vi "Scale Controls.vi"(7 "rules":string, 8 "error in (no error)":errorcluster, 9 "pane size":T3, 10 "Decorations on Pane":refnum<vi>[](array[refnum]), 11 "Controls on Pane":refnum<vi>[](array[refnum])) -> (0 "error out":errorcluster)   [LabVIEW 2020]
doc: "Simple and schmutzig VI that will scale controls and labeled decorations by delta change of pane size.\nUsage: put in multiline string with rules:\nmy control name a [edge:LRTB]\nmy control name b [edge:LRB]\n...\n\nwhere edge:LRTB defines edges to be sticked to pane. LR - scale horizontaly, R - no scale, move object only, TB - scale vertically, B - just stick object to bottom, no scaling...\nWhen using for decorations, name them first with script 'Set Decoration Label'!"
uses:
  <vilib>/Utility/miscctls.llb/LVRectTypeDef.ctl
  Scale Controls List.ctl
  Scale Controls Record.ctl
  <vilib>/regexp/Match Regular Expression.xnode
panel:
  in  "lists":T1[](array[typedef])
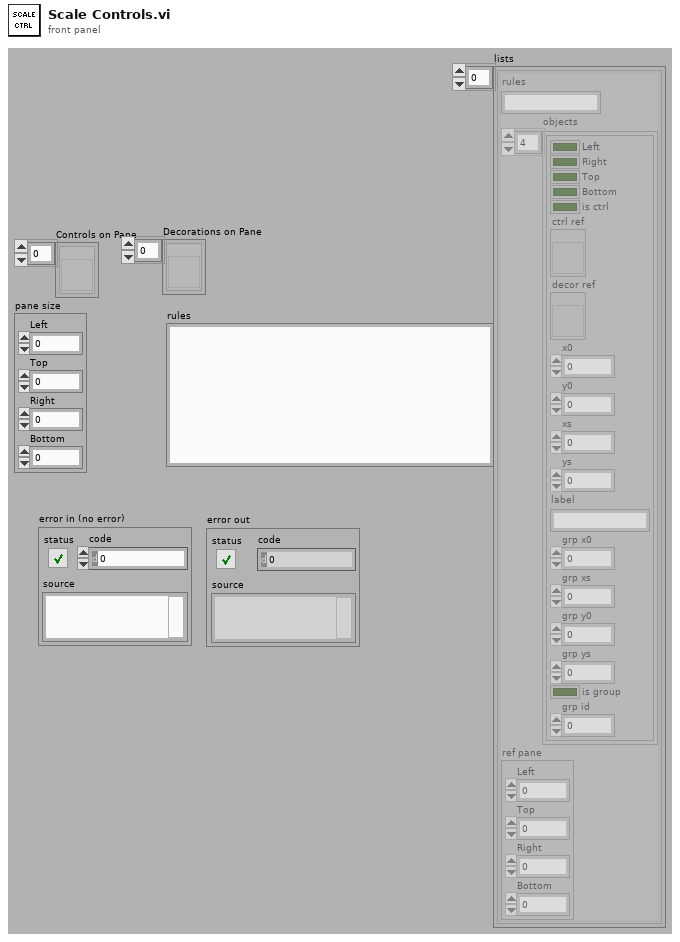
[diagram p1: front panel]
types:
  T1 = typedef "Scale Controls List.ctl" = cluster{"rules":string, "objects":T2[], "ref pane":T3}
  T2 = typedef "Scale Controls Record.ctl" = cluster{"Left":bool, "Right":bool, "Top":bool, "Bottom":bool, "is ctrl":bool, "ctrl ref":refnum<vi>, "decor ref":refnum<vi>, "x0":i32, "y0":i32, "xs":i32, "ys":i32, "label":string, "grp x0":i32, "grp xs":i32, "grp y0":i32, "grp ys":i32, "is group":bool, "grp id":i32}
  T3 = typedef "LVRectTypeDef.ctl" = cluster{"Left":i16, "Top":i16, "Right":i16, "Bottom":i16}
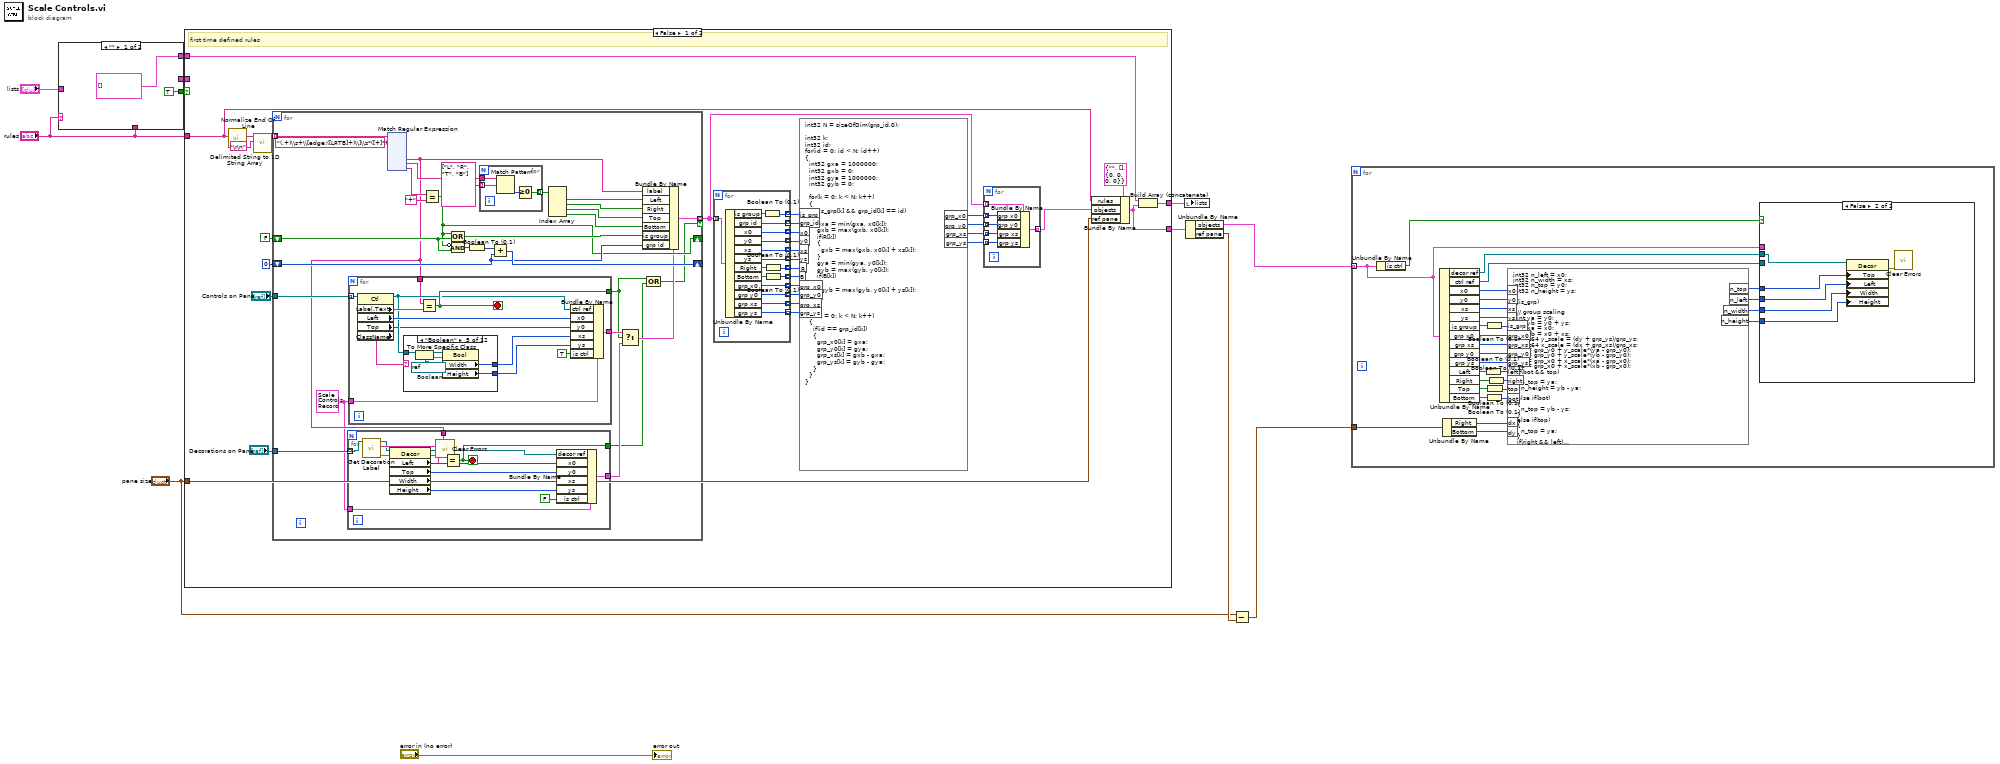
[diagram p0: block diagram]
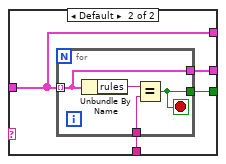
[diagram p2: hidden frame]
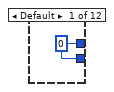
[diagram p3: hidden frame]
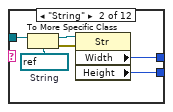
[diagram p4: hidden frame]
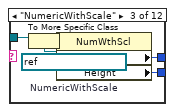
[diagram p5: hidden frame]
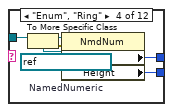
[diagram p6: hidden frame]
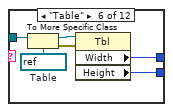
[diagram p7: hidden frame]
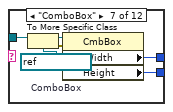
[diagram p8: hidden frame]
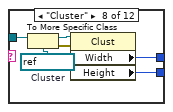
[diagram p9: hidden frame]
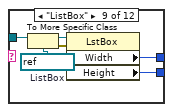
[diagram p10: hidden frame]
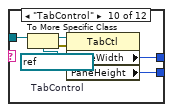
[diagram p11: hidden frame]
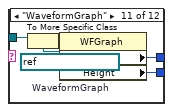
[diagram p12: hidden frame]
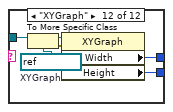
[diagram p13: hidden frame]
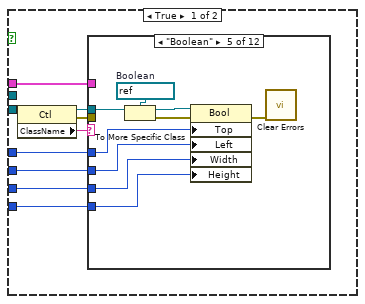
[diagram p15: hidden frame]
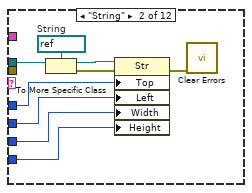
[diagram p17: hidden frame]
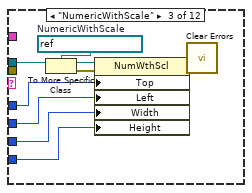
[diagram p18: hidden frame]
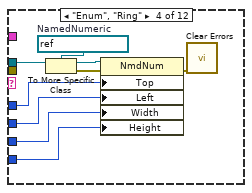
[diagram p19: hidden frame]
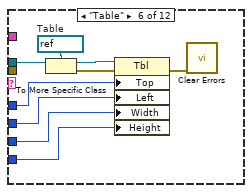
[diagram p20: hidden frame]
diagram:
  n1 = case shown="\"\"" "rules" {
    tunnel: [TRUE w18] -> w11
    tunnel: [_ w17] -> w9
    tunnel: "rules" -> [_ w16]
    tunnel: [T1[] [] ("lists") w15] -> w7
    tunnel: "lists" -> [_ w15]
    frame "" {
    }
    frame Default {
      n2 = for {
        tunnel: w15 -> [w19] mode=indexing
        tunnel: w16 -> [w21]
        tunnel: [w20] -> w18
        tunnel: [w19] -> w17
        stop <- w20 stop-if-true
        n3 = Unbundle By Name(w19) -> ("rules"=w22:string)
        n4 = Equal?(x=w22, y=w21) -> (x = y?=w20:bool)
      }
    }
  }
  n5 = case shown="False" w11 {
    tunnel: "rules" -> [w48 _]
    tunnel: w7 -> [w47 w322]
    tunnel: [w46 w322] -> w10
    tunnel: [w45 w323] -> w8
    tunnel: w9 -> [_ w323]
    tunnel: "pane size" -> [w44 _]
    frame False {
      # "first time defined rules"
      n6 = call <vilib>:"Normalize End Of Line.vi"("string in"=w48) -> ("string out"=w51:string)  [unwired: 7 in]
      n7 = call <vilib>:"Delimited String to 1D String Array.vi"("delimiter"="\r\n", "delimited string"=w51) -> ("string array"=w52:string[])  [unwired: 9 in]
      n8 = for {
        tunnel: w52 -> [w104] mode=indexing
        tunnel: [w94] -> w30 mode=indexing if=w76
        tunnel: "Controls on Pane" -> [w95]
        shift-right: [w85] -> _
        shift-left: FALSE -> [w91]
        shift-right: [w88] -> _
        shift-left: 0 -> [w87]
        tunnel: "Decorations on Pane" -> [w84]
        w82 = T2 {"Left"=FALSE, "Right"=FALSE, "Top"=FALSE, "Bottom"=FALSE, "is ctrl"=FALSE, "ctrl ref"=refnum, "decor ref"=refnum, "x0"=0, "y0"=0, "xs"=0, "ys"=0, "label"="", "grp x0"=0, "grp xs"=0, "grp y0"=0, "grp ys"=0, "is group"=FALSE, "grp id"=0} ("object")
        n9 = xnode "Match Regular Expression"("input string"=w104, "regular expression"="(.+)\\s+\\[edge:([LRTB]+)\\]\\s*([+]*)") -> ("submatch 1"=w83:string, "submatch 2"=w102:string, "submatch 3"=w93:string)  [unwired: 4 in, 5 out]
        n10 = for {
          tunnel: w84 -> [w108] mode=indexing
          tunnel: w83 -> [w115]
          tunnel: w82 -> [w114]
          tunnel: [w117] -> w80
          tunnel: [w116] -> w77
          stop <- w116 stop-if-true
          n11 = call "Get Decoration Label.vi"("Decor Refnum"=w108) -> ("error out"=w109:errorcluster, "Label"=w110:string, "dup Decor Refnum"=w107:refnum<vi>)  [unwired: 4 in]
          n12 = property class="Decor"(reference=w107, error in=w109) -> (reference out=w106:refnum<vi>, error out=w105:errorcluster, "Left"=w119:i32, "Top"=w113:i32, "Width"=w112:u32, "Height"=w111:u32)
          n13 = call <vilib>:"Clear Errors.vi"("error in (no error)"=w105) -> ()  [unwired: 5 in, 2 out]
          n14 = Equal?(x=w115, y=w110) -> (x = y?=w116:bool)
          n15 = Bundle By Name(cluster=w114, "decor ref"=w106, "x0"=w119, "y0"=w113, "xs"=w112, "ys"=w111, "is ctrl"=FALSE) -> (w117:T2)
        }
        n16 = for {
          tunnel: w95 -> [w132] mode=indexing
          tunnel: w83 -> [w124]
          tunnel: w82 -> [w122]
          tunnel: [w128] -> w81
          tunnel: [w127] -> w78
          stop <- w127 stop-if-true
          n17 = property class="Ctl"(reference=w132) -> (reference out=w126:refnum<vi>, "Label.Text"=w131:string, "Left"=w130:i32, "Top"=w120:i32, "ClassName"=w125:string)  [unwired: 1 in, 1 out]
          n18 = case shown="\"Boolean\"" w125 {
            tunnel: w126 -> [_ w136 w142 w148 w154 w160 w166 w172 w178 w184 w190 w196]
            tunnel: [w133 w135 w141 w147 w153 w159 w165 w171 w177 w183 w189 w195] -> w123
            tunnel: [w133 w134 w140 w146 w152 w158 w164 w170 w176 w182 w188 w194] -> w121
            frame Default {
              w133 = u32 0 ("Width")
            }
            frame "String" {
              w139 = refnum<vi> refnum  # String
              n19 = To More Specific Class(target class=w139, reference=w136) -> (specific class reference=w137:refnum<vi>, error out=w138:errorcluster)  [unwired: 1 in]
              n20 = property class="Str"(reference=w137, error in=w138) -> ("Width"=w135:u32, "Height"=w134:u32)  [unwired: 2 out]
            }
            frame "NumericWithScale" {
              w145 = refnum<vi> refnum  # NumericWithScale
              n21 = To More Specific Class(target class=w145, reference=w142) -> (specific class reference=w143:refnum<vi>, error out=w144:errorcluster)  [unwired: 1 in]
              n22 = property class="NumWthScl"(reference=w143, error in=w144) -> ("Width"=w141:u32, "Height"=w140:u32)  [unwired: 2 out]
            }
            frame "Enum", "Ring" {
              w151 = refnum<vi> refnum  # NamedNumeric
              n23 = To More Specific Class(target class=w151, reference=w148) -> (specific class reference=w149:refnum<vi>, error out=w150:errorcluster)  [unwired: 1 in]
              n24 = property class="NmdNum"(reference=w149, error in=w150) -> ("Width"=w147:u32, "Height"=w146:u32)  [unwired: 2 out]
            }
            frame "Boolean" {
              w157 = refnum<vi> refnum  # Boolean
              n25 = To More Specific Class(target class=w157, reference=w154) -> (specific class reference=w155:refnum<vi>, error out=w156:errorcluster)  [unwired: 1 in]
              n26 = property class="Bool"(reference=w155, error in=w156) -> ("Width"=w153:u32, "Height"=w152:u32)  [unwired: 2 out]
            }
            frame "Table" {
              w163 = refnum<vi> refnum  # Table
              n27 = To More Specific Class(target class=w163, reference=w160) -> (specific class reference=w161:refnum<vi>, error out=w162:errorcluster)  [unwired: 1 in]
              n28 = property class="Tbl"(reference=w161, error in=w162) -> ("Width"=w159:u32, "Height"=w158:u32)  [unwired: 2 out]
            }
            frame "ComboBox" {
              w169 = refnum<vi> refnum  # ComboBox
              n29 = To More Specific Class(target class=w169, reference=w166) -> (specific class reference=w167:refnum<vi>, error out=w168:errorcluster)  [unwired: 1 in]
              n30 = property class="CmbBox"(reference=w167, error in=w168) -> ("Width"=w165:u32, "Height"=w164:u32)  [unwired: 2 out]
            }
            frame "Cluster" {
              w175 = refnum<vi> refnum  # Cluster
              n31 = To More Specific Class(target class=w175, reference=w172) -> (specific class reference=w173:refnum<vi>, error out=w174:errorcluster)  [unwired: 1 in]
              n32 = property class="Clust"(reference=w173, error in=w174) -> ("Width"=w171:u32, "Height"=w170:u32)  [unwired: 2 out]
            }
            frame "ListBox" {
              w181 = refnum<vi> refnum  # ListBox
              n33 = To More Specific Class(target class=w181, reference=w178) -> (specific class reference=w179:refnum<vi>, error out=w180:errorcluster)  [unwired: 1 in]
              n34 = property class="LstBox"(reference=w179, error in=w180) -> ("Width"=w177:u32, "Height"=w176:u32)  [unwired: 2 out]
            }
            frame "TabControl" {
              w187 = refnum<vi> refnum  # TabControl
              n35 = To More Specific Class(target class=w187, reference=w184) -> (specific class reference=w185:refnum<vi>, error out=w186:errorcluster)  [unwired: 1 in]
              n36 = property class="TabCtl"(reference=w185, error in=w186) -> ("PaneWidth"=w183:u32, "PaneHeight"=w182:u32)  [unwired: 2 out]
            }
            frame "WaveformGraph" {
              w193 = refnum<vi> refnum  # WaveformGraph
              n37 = To More Specific Class(target class=w193, reference=w190) -> (specific class reference=w191:refnum<vi>, error out=w192:errorcluster)  [unwired: 1 in]
              n38 = property class="WFGraph"(reference=w191, error in=w192) -> ("Width"=w189:u32, "Height"=w188:u32)  [unwired: 2 out]
            }
            frame "XYGraph" {
              w199 = refnum<vi> refnum  # XYGraph
              n39 = To More Specific Class(target class=w199, reference=w196) -> (specific class reference=w197:refnum<vi>, error out=w198:errorcluster)  [unwired: 1 in]
              n40 = property class="XYGraph"(reference=w197, error in=w198) -> ("Width"=w195:u32, "Height"=w194:u32)  [unwired: 2 out]
            }
          }
          n41 = Equal?(x=w124, y=w131) -> (x = y?=w127:bool)
          n42 = Bundle By Name(cluster=w122, "ctrl ref"=w126, "x0"=w130, "y0"=w120, "xs"=w123, "ys"=w121, "is ctrl"=TRUE) -> (w128:T2)
        }
        n43 = Equal?(x=w93, y="+") -> (x = y?=w85:bool)
        n44 = Compound Arithmetic op=OR(w85, w91) -> (w86:bool)
        n45 = Compound Arithmetic op=AND(invert w85, w91) -> (w90:bool)
        n46 = Boolean To (0,1)(Boolean=w90) -> (0, 1=w89:i16)
        n47 = for {
          tunnel: w102 -> [w203]
          tunnel: string[] ["L", "R", "T", "B"] -> [w202] mode=indexing
          tunnel: [w200] -> w100 mode=indexing
          n48 = Match Pattern(string=w203, regular expression=w202) -> (offset past match=w201:i32)  [unwired: 1 in, 3 out]
          n49 = Greater Or Equal To 0?(x=w201) -> (x >= 0?=w200:bool)
        }
        n50 = Add(x=w89, y=w87) -> (x+y=w88:i32)
        n51 = Index Array(array=w100) -> (element #1=w99:bool, element #2=w98:bool, element #3=w97:bool, element #4=w96:bool)  [unwired: 4 in]
        n52 = Select(t=w81, s=w78, f=w80) -> (s? t:f=w79:T2)
        n53 = Bundle By Name(cluster=w79, "label"=w83, "Left"=w99, "Right"=w98, "Top"=w97, "Bottom"=w96, "is group"=w86, "grp id"=w87) -> (w94:T2)
        n54 = Compound Arithmetic op=OR(w78, w77) -> (w76:bool)
      }
      n55 = for {
        tunnel: w30 -> [w75] mode=indexing
        tunnel: [w73] -> w41 mode=indexing
        tunnel: [w72] -> w24 mode=indexing
        tunnel: [w71] -> w40 mode=indexing
        tunnel: [w70] -> w39 mode=indexing
        tunnel: [w69] -> w38 mode=indexing
        tunnel: [w68] -> w37 mode=indexing
        tunnel: [w66] -> w36 mode=indexing
        tunnel: [w64] -> w35 mode=indexing
        tunnel: [w63] -> w34 mode=indexing
        tunnel: [w62] -> w33 mode=indexing
        tunnel: [w61] -> w32 mode=indexing
        tunnel: [w60] -> w31 mode=indexing
        n56 = Unbundle By Name(w75) -> ("is group"=w74:bool, "grp id"=w73:i32, "x0"=w71:i32, "y0"=w70:i32, "xs"=w69:i32, "ys"=w68:i32, "Right"=w67:bool, "Bottom"=w65:bool, "grp x0"=w63:i32, "grp y0"=w62:i32, "grp xs"=w61:i32, "grp ys"=w60:i32)
        n57 = Boolean To (0,1)(Boolean=w74) -> (0, 1=w72:i16)
        n58 = Boolean To (0,1)(Boolean=w67) -> (0, 1=w66:i16)
        n59 = Boolean To (0,1)(Boolean=w65) -> (0, 1=w64:i16)
      }
      n60 = formula code="int32 N = sizeOfDim(grp_id,0);\n\nint32 k;\nint32 id;\nfor(id = 0; id < N; id++)\n{\n  int32 gxa = 1000000;\n  int32 gxb = 0;\n  int32 gya = 1000000;\n  int32 gyb = 0;\n\n  for(k = 0; k < N; k++)\n  {\n    if(is_grp[k] && grp_id[k] == id)\n    {\n      gxa = min(gxa, x0[k]);\n      gxb = max(gxb, x0[k]);\n      if(R[k])\n      {\n        gxb = max(gxb, x0[k] + xs[k]);\n      }\n      gya = min(gya, y0[k]);\n      gyb = max(gyb, y0[k]);\n      if(B[k])\n      {\n        gyb = max(gyb, y0[k] + ys[k]);\n      }\n    }\n  }\n  for(k = 0; k < N; k++)\n  {\n    if(id == grp_id[k])\n    {\n      grp_x0[k] = gxa;\n      grp_y0[k] = gya;\n      grp_xs[k] = gxb - gxa;\n      grp_ys[k] = gyb - gya;\n    }\n  }\n}"("is_grp"=w24, "grp_id"=w41, "x0"=w40, "y0"=w39, "xs"=w38, "ys"=w37, "R"=w36, "B"=w35, "grp_x0"=w34, "grp_y0"=w33, "grp_xs"=w32, "grp_ys"=w31) -> ("grp_x0"=w29:i32[], "grp_y0"=w28:i32[], "grp_xs"=w27:i32[], "grp_ys"=w26:i32[])
      n61 = for {
        tunnel: w30 -> [w59] mode=indexing
        tunnel: w29 -> [w58] mode=indexing
        tunnel: w28 -> [w57] mode=indexing
        tunnel: w27 -> [w56] mode=indexing
        tunnel: w26 -> [w55] mode=indexing
        tunnel: [w54] -> w25 mode=indexing
        n62 = Bundle By Name(cluster=w59, "grp x0"=w58, "grp y0"=w57, "grp xs"=w56, "grp ys"=w55) -> (w54:T2)
      }
      n63 = Bundle By Name(cluster=T1 {"rules"="", "objects"=[], "ref pane"={"Left"=0, "Top"=0, "Right"=0, "Bottom"=0}} ("obj list"), "rules"=w48, "objects"=w25, "ref pane"=w44) -> (w45:T1)
      n64 = Build Array (concatenate)(w47, w45) -> (w46:T1[])
    }
    frame True {
      # "old rules found"
    }
  }
  n65 = local write "lists"(w10) -> ()
  n66 = Unbundle By Name(w8) -> ("objects"=w6:T2[], "ref pane"=w5:T3)
  n67 = Subtract(x="pane size", y=w5) -> (x-y=w3:T3)
  n68 = for {
    tunnel: w3 -> [w352]
    tunnel: w6 -> [w351] mode=indexing
    n69 = Unbundle By Name(w351) -> ("is ctrl"=w325:bool)
    n70 = Unbundle By Name(w351) -> ("decor ref"=w324:refnum<vi>, "ctrl ref"=w350:refnum<vi>, "x0"=w349:i32, "y0"=w348:i32, "xs"=w347:i32, "ys"=w346:i32, "is group"=w345:bool, "grp x0"=w343:i32, "grp xs"=w341:i32, "grp y0"=w342:i32, "grp ys"=w340:i32, "Left"=w339:bool, "Right"=w337:bool, "Top"=w335:bool, "Bottom"=w333:bool)
    n71 = Unbundle By Name(w352) -> ("Right"=w327:i16, "Bottom"=w326:i16)
    n72 = Boolean To (0,1)(Boolean=w339) -> (0, 1=w338:i16)
    n73 = Boolean To (0,1)(Boolean=w345) -> (0, 1=w344:i16)
    n74 = Boolean To (0,1)(Boolean=w333) -> (0, 1=w332:i16)
    n75 = Boolean To (0,1)(Boolean=w335) -> (0, 1=w334:i16)
    n76 = Boolean To (0,1)(Boolean=w337) -> (0, 1=w336:i16)
    n77 = formula code="int32 n_left = x0;\nint32 n_width = xs;\nint32 n_top = y0;\nint32 n_height = ys;\n\nif(is_grp)\n{\n  // group scaling\n  int ya = y0;\n  int yb = y0 + ys;\n  int xa = x0;\n  int xb = x0 + xs;\n  float64 y_scale = (dy + grp_ys)/grp_ys;\n  float64 x_scale = (dx + grp_xs)/grp_xs;\n  ya = grp_y0 + y_scale*(ya - grp_y0);\n  yb = grp_y0 + y_scale*(yb - grp_y0);\n  xa = grp_x0 + x_scale*(xa - grp_x0);\n  xb = grp_x0 + x_scale*(xb - grp_x0);\n  if(bot && top)\n  {\n    n_top = ya;\n    n_height = yb - ya;\n  }\n  else if(bot)\n  {\n    n_top = yb - ys;\n  }\n  else if(top)\n  {\n    n_top = ya;\n  }\n  if(right && left)\n  {\n    n_left = xa;\n    n_width = xb - xa;\n  }\n  else if(right)\n  {\n    n_left = xb - xs;\n  }\n  else if(left)\n  {\n    n_left = xa;\n  }\n}\nelse\n{\n  if(bot && top)\n    n_height = ys + dy;\n  if(bot && !top)\n    n_top = y0 + dy;\n  if(right && left)\n    n_width = xs + dx;\n  if(right && !left)\n    n_left = x0 + dx;\n}"("x0"=w349, "y0"=w348, "xs"=w347, "ys"=w346, "is_grp"=w344, "grp_x0"=w343, "grp_y0"=w342, "grp_xs"=w341, "grp_ys"=w340, "left"=w338, "right"=w336, "top"=w334, "bot"=w332, "dx"=w327, "dy"=w326) -> ("n_top"=w331:i32, "n_left"=w330:i32, "n_width"=w329:i32, "n_height"=w328:i32)
    n78 = case shown="False" w325 {
      tunnel: w351 -> [w361 _]
      tunnel: w350 -> [w358 _]
      tunnel: w331 -> [w356 w464]
      tunnel: w330 -> [w355 w463]
      tunnel: w329 -> [w354 w462]
      tunnel: w328 -> [w353 w461]
      tunnel: w324 -> [_ w459]
      frame True {
        n79 = property class="Ctl"(reference=w358) -> (reference out=w360:refnum<vi>, error out=w357:errorcluster, "ClassName"=w359:string)  [unwired: 1 in]
        n80 = case shown="\"Boolean\"" w359 {
          tunnel: w360 -> [_ w370 w379 w388 w397 w406 w415 w424 w433 w440 w449 w458]
          tunnel: w361 -> [_ _ _ _ _ _ _ _ _ _ _ _]
          tunnel: w357 -> [_ _ _ _ _ _ _ _ _ _ _ _]
          tunnel: w356 -> [_ w366 w375 w384 w393 w402 w411 w420 w429 w436 w445 w454]
          tunnel: w355 -> [_ w365 w374 w383 w392 w401 w410 w419 w428 w435 w444 w453]
          tunnel: w354 -> [_ w364 w373 w382 w391 w400 w409 w418 w427 _ w443 w452]
          tunnel: w353 -> [_ w363 w372 w381 w390 w399 w408 w417 w426 _ w442 w451]
          frame Default {
          }
          frame "String" {
            w368 = refnum<vi> refnum  # String
            n81 = To More Specific Class(target class=w368, reference=w370) -> (specific class reference=w369:refnum<vi>, error out=w367:errorcluster)  [unwired: 1 in]
            n82 = property class="Str"(reference=w369, error in=w367, "Top"=w366, "Left"=w365, "Width"=w364, "Height"=w363) -> (error out=w362:errorcluster)  [unwired: 1 out]
            n83 = call <vilib>:"Clear Errors.vi"("error in (no error)"=w362) -> ()  [unwired: 5 in, 2 out]
          }
          frame "NumericWithScale" {
            w377 = refnum<vi> refnum  # NumericWithScale
            n84 = To More Specific Class(target class=w377, reference=w379) -> (specific class reference=w378:refnum<vi>, error out=w376:errorcluster)  [unwired: 1 in]
            n85 = property class="NumWthScl"(reference=w378, error in=w376, "Top"=w375, "Left"=w374, "Width"=w373, "Height"=w372) -> (error out=w371:errorcluster)  [unwired: 1 out]
            n86 = call <vilib>:"Clear Errors.vi"("error in (no error)"=w371) -> ()  [unwired: 5 in, 2 out]
          }
          frame "Enum", "Ring" {
            w386 = refnum<vi> refnum  # NamedNumeric
            n87 = To More Specific Class(target class=w386, reference=w388) -> (specific class reference=w387:refnum<vi>, error out=w385:errorcluster)  [unwired: 1 in]
            n88 = property class="NmdNum"(reference=w387, error in=w385, "Top"=w384, "Left"=w383, "Width"=w382, "Height"=w381) -> (error out=w380:errorcluster)  [unwired: 1 out]
            n89 = call <vilib>:"Clear Errors.vi"("error in (no error)"=w380) -> ()  [unwired: 5 in, 2 out]
          }
          frame "Boolean" {
            w395 = refnum<vi> refnum  # Boolean
            n90 = To More Specific Class(target class=w395, reference=w397) -> (specific class reference=w396:refnum<vi>, error out=w394:errorcluster)  [unwired: 1 in]
            n91 = property class="Bool"(reference=w396, error in=w394, "Top"=w393, "Left"=w392, "Width"=w391, "Height"=w390) -> (error out=w389:errorcluster)  [unwired: 1 out]
            n92 = call <vilib>:"Clear Errors.vi"("error in (no error)"=w389) -> ()  [unwired: 5 in, 2 out]
          }
          frame "Table" {
            w404 = refnum<vi> refnum  # Table
            n93 = To More Specific Class(target class=w404, reference=w406) -> (specific class reference=w405:refnum<vi>, error out=w403:errorcluster)  [unwired: 1 in]
            n94 = property class="Tbl"(reference=w405, error in=w403, "Top"=w402, "Left"=w401, "Width"=w400, "Height"=w399) -> (error out=w398:errorcluster)  [unwired: 1 out]
            n95 = call <vilib>:"Clear Errors.vi"("error in (no error)"=w398) -> ()  [unwired: 5 in, 2 out]
          }
          frame "TabControl" {
            w413 = refnum<vi> refnum  # TabControl
            n96 = To More Specific Class(target class=w413, reference=w415) -> (specific class reference=w414:refnum<vi>, error out=w412:errorcluster)  [unwired: 1 in]
            n97 = property class="TabCtl"(reference=w414, error in=w412, "Top"=w411, "Left"=w410, "PaneWidth"=w409, "PaneHeight"=w408) -> (error out=w407:errorcluster)  [unwired: 1 out]
            n98 = call <vilib>:"Clear Errors.vi"("error in (no error)"=w407) -> ()  [unwired: 5 in, 2 out]
          }
          frame "ComboBox" {
            w422 = refnum<vi> refnum  # ComboBox
            n99 = To More Specific Class(target class=w422, reference=w424) -> (specific class reference=w423:refnum<vi>, error out=w421:errorcluster)  [unwired: 1 in]
            n100 = property class="CmbBox"(reference=w423, error in=w421, "Top"=w420, "Left"=w419, "Width"=w418, "Height"=w417) -> (error out=w416:errorcluster)  [unwired: 1 out]
            n101 = call <vilib>:"Clear Errors.vi"("error in (no error)"=w416) -> ()  [unwired: 5 in, 2 out]
          }
          frame "ListBox" {
            w431 = refnum<vi> refnum  # ListBox
            n102 = To More Specific Class(target class=w431, reference=w433) -> (specific class reference=w432:refnum<vi>, error out=w430:errorcluster)  [unwired: 1 in]
            n103 = property class="LstBox"(reference=w432, error in=w430, "Top"=w429, "Left"=w428, "Width"=w427, "Height"=w426) -> (error out=w425:errorcluster)  [unwired: 1 out]
            n104 = call <vilib>:"Clear Errors.vi"("error in (no error)"=w425) -> ()  [unwired: 5 in, 2 out]
          }
          frame "Cluster" {
            w438 = refnum<vi> refnum  # Cluster
            n105 = To More Specific Class(target class=w438, reference=w440) -> (specific class reference=w439:refnum<vi>, error out=w437:errorcluster)  [unwired: 1 in]
            n106 = property class="Clust"(reference=w439, error in=w437, "Top"=w436, "Left"=w435) -> (error out=w434:errorcluster)  [unwired: 1 out]
            n107 = call <vilib>:"Clear Errors.vi"("error in (no error)"=w434) -> ()  [unwired: 5 in, 2 out]
          }
          frame "XYGraph" {
            w447 = refnum<vi> refnum  # XYGraph
            n108 = To More Specific Class(target class=w447, reference=w449) -> (specific class reference=w448:refnum<vi>, error out=w446:errorcluster)  [unwired: 1 in]
            n109 = property class="XYGraph"(reference=w448, error in=w446, "Top"=w445, "Left"=w444, "Width"=w443, "Height"=w442) -> (error out=w441:errorcluster)  [unwired: 1 out]
            n110 = call <vilib>:"Clear Errors.vi"("error in (no error)"=w441) -> ()  [unwired: 5 in, 2 out]
          }
          frame "WaveformGraph" {
            w456 = refnum<vi> refnum  # WaveformGraph
            n111 = To More Specific Class(target class=w456, reference=w458) -> (specific class reference=w457:refnum<vi>, error out=w455:errorcluster)  [unwired: 1 in]
            n112 = property class="WFGraph"(reference=w457, error in=w455, "Top"=w454, "Left"=w453, "Width"=w452, "Height"=w451) -> (error out=w450:errorcluster)  [unwired: 1 out]
            n113 = call <vilib>:"Clear Errors.vi"("error in (no error)"=w450) -> ()  [unwired: 5 in, 2 out]
          }
        }
      }
      frame False {
        n114 = property class="Decor"(reference=w459, "Top"=w464, "Left"=w463, "Width"=w462, "Height"=w461) -> (error out=w460:errorcluster)  [unwired: 1 in, 1 out]
        n115 = call <vilib>:"Clear Errors.vi"("error in (no error)"=w460) -> ()  [unwired: 5 in, 2 out]
      }
    }
  }
  "error out" <- "error in (no error)"
